vi "SPI Split Control Lines.vi"(11 "SPCR":u16) -> (0 "Sample on trailing edge (Phase)?":bool, 1 "Falling edge leads (Polarity)?":bool, 2 "LSB first?":bool, 3 "Frame Length":T1, 4 "Slave?":bool, 5 "Clock Select":T2)   [LabVIEW 2014]
uses:
  SPI Clock Select.ctl
  SPI Frame Length.ctl
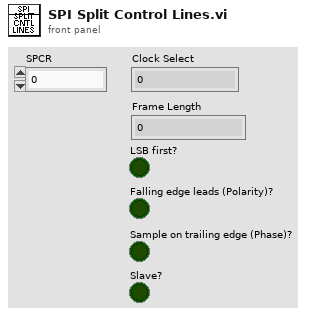
[diagram p1: front panel]
types:
  T1 = typedef "SPI Frame Length.ctl" = fxp<+,4,4>
  T2 = typedef "SPI Clock Select.ctl" = fxp<+,2,2>
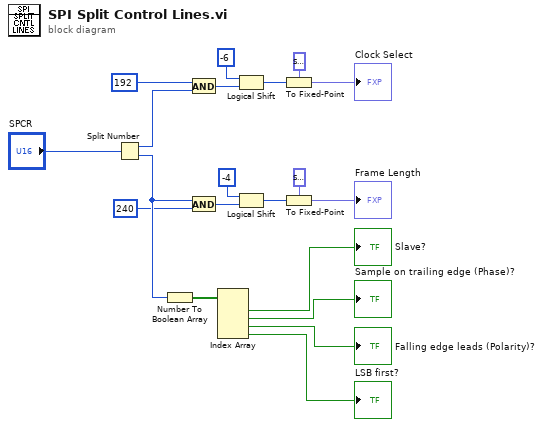
[diagram p0: block diagram]
diagram:
  n1 = Split Number(x="SPCR") -> (hi(x)=w11:u8, lo(x)=w16:u8)
  n2 = Number To Boolean Array(number=w16) -> (Boolean array=w17:bool[])
  n3 = And(x=u8 192 ("y"), y=w11) -> (x .and. y?=w9:u8)
  n4 = And(x=w16, y=u8 240) -> (x .and. y?=w14:u8)
  n5 = Index Array(array=w17) -> (element #1=→"Slave?":bool, element #2=→"Sample on trailing edge (Phase)?":bool, element #3=→"Falling edge leads (Polarity)?":bool, element #4=→"LSB first?":bool)  [unwired: 4 in]
  n6 = Logical Shift(y=i8 -6, x=w9) -> (x << y=w7:u8)
  n7 = Logical Shift(y=i8 -4, x=w14) -> (x << y=w12:u8)
  n8 = To Fixed-Point(fixed-point type=T2 0.0 ("Clock Select"), number=w7) -> (fixed-point=→"Clock Select":T2)
  n9 = To Fixed-Point(fixed-point type=T1 0.0 ("Frame Length"), number=w12) -> (fixed-point=→"Frame Length":T1)
